vi "Controller Write FXP22.4.vi"(8 "Error In":errorcluster, 10 "Values":fxp<+/-,22,4>[](array[numeric]), 11 "Variables":refnum<k21>[](array[refnum])) -> (0 "Error Out":errorcluster)   [LabVIEW 2011, in "Controller VIs.lvlib"]
doc: "Writes a vector of fixed-Point <+/-,20,5> I/O variables."
uses:
  Controller VIs.lvlib
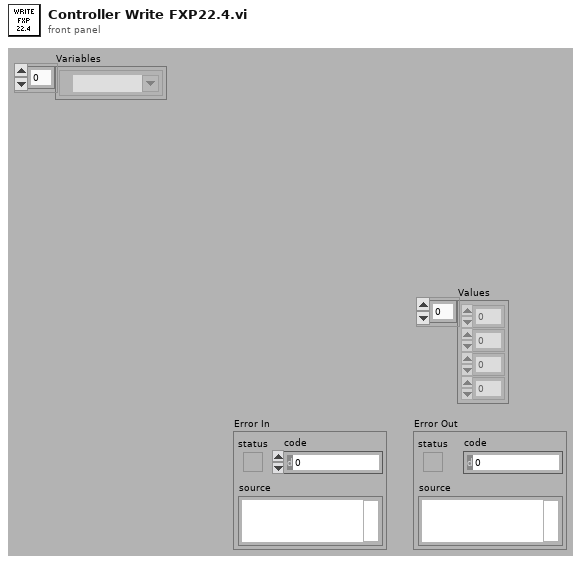
[diagram p1: front panel]
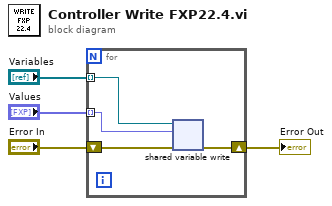
[diagram p0: block diagram]
diagram:
  n1 = for {
    tunnel: "Values" -> [w6] mode=indexing
    shift-right: [w7] -> w3
    shift-left: "Error In" -> [w8]
    tunnel: "Variables" -> [w5] mode=indexing
    n2 = shared-variable-write(w5, w8, w6) -> (w7:errorcluster)  [unwired: 1 out]
  }
  "Error Out" <- w3
